vi "interfaz-grafica - Control Mouse.vi"() -> ()   [LabVIEW 2024]
uses:
  TG JD - running/TG Juan Diego/Documentos de Labview/160620 Optotune Lens Driver 4 Labview package/Hello Optotune Lens (30.06.2015)/Calibration.ctl
  <vilib>/vision/Avi.llb/IMAQ AVI2 Refnum.ctl
  <vilib>/Instr/_visa.llb/VISA Configure Serial Port (Instr).vi
  <vilib>/Utility/file.llb/Write Delimited Spreadsheet (string).vi
  <vilib>/Utility/file.llb/Read Delimited Spreadsheet (string).vi
  <vilib>/Utility/inputDevices.llb/mouseAcquire.vi
  <vilib>/Utility/inputDevices.llb/closeMouse.vi
  <vilib>/vision/NI_Vision_Development_Module.lvlib
panel:
  out "Path Pot Inicial IZQUIERDA":path
  out "Path Pot Inicial DERECHA":path
  out "PI_I":dbl(slide) scale=-3.0..3.0
  out "PI_D":dbl(slide) scale=-3.0..3.0
  in  "stop 7":bool
  in  "CONTROL":bool
  out "axis info":T1
  in  "stop 6":bool
  out "Vertical":i32
  out "Dioptrias Finales":dbl
  out "AVI Refnum":T2
  in  "stop 5":bool
  out "Boolean":bool
  out "Usuario 3":string(combo)
  out "Usuario 2":string(combo)
  out "USUARIO 2":string caption="USUARIO"
  out "Path Video":path
  out "Path Potencia Optica D":path
  out "Path Potencia Optica I":path
  in  "stop":bool
  out "Array 2":dbl[](array[numeric])
  out "Array":dbl[](array[numeric])
  out "Path DATOS":path
  in  "stop 2":bool
  out "Path":path=path "C:/Users/willi/GITHUB/TG/OBJ 2 - RECOLECCION DE DATOS/registro-usuarios.csv"
  out "error out":errorcluster
  in  "Tab Control":enum32{"Experimento", "Configuración"}(tab)
  in  "ADQUIRIR":bool
  in  "DETENER":bool
  out "DPT  IZQ":dbl
  out "DPT  DER":dbl
  out "Potencia  Ojo Derecho":dbl[](graph)
  out "ROI (Ojo)":T3(plugin-control)
  out "Path ADQUISICION":path
  in  "Potencia inicial lente derecho":dbl(slide) scale=-3.0..3.0
  in  "Potencia inicial lente izquierdo":dbl(slide) scale=-3.0..3.0
  out "Full Image":T3(plugin-control)
  in  "VISA resource name 3":refnum<visa-resource-name>
  in  "Tab Control 2":T4(tab)
  in  "Usuario":string(combo)
  in  "registrarButtom":bool
  in  "Cluster":T5 {"Fecha de nacimiento" format="%<%x>T"}
  out "Nuevo Usuario":i32
  out "USUARIO":string
  in  "VISA resource name 4":refnum<visa-resource-name>
  out "error out 4":errorcluster
  out "error out 3":errorcluster
  in  "stop 4":bool
  in  "error in (no error) 3":errorcluster
  in  "error in (no error) 4":errorcluster
  in  "stop 3":bool
  out "VISA resource name out 2":string
  out "Command to Port":string
  out "Data":string
  out "OK":bool
  out "Calibration 2":T6 {"Max Current A" format="%#_g mA"; "Max Current B" format="%#_g mA"; "UCL A" format="%#_g mA"; "LCL A" format="%#_g mA"; "UCL B" format="%#_g mA"; "LCL B" format="%#_g mA"}
  out "VISA resource name out":string
  out "ID":u16
  in  "Calibration":T6={"Max Current A"=293.0, "Max Current B"=293.0, "UCL A"=300.0, "UCL B"=300.0, "LCL A"=0.0, "LCL B"=0.0} {"Max Current A" format="%#_g mA"; "Max Current B" format="%#_g mA"; "UCL A" format="%#_g mA"; "LCL A" format="%#_g mA"; "UCL B" format="%#_g mA"; "LCL B" format="%#_g mA"}
  # "Seleccione la Region de Interes (ROI. el ojo)"
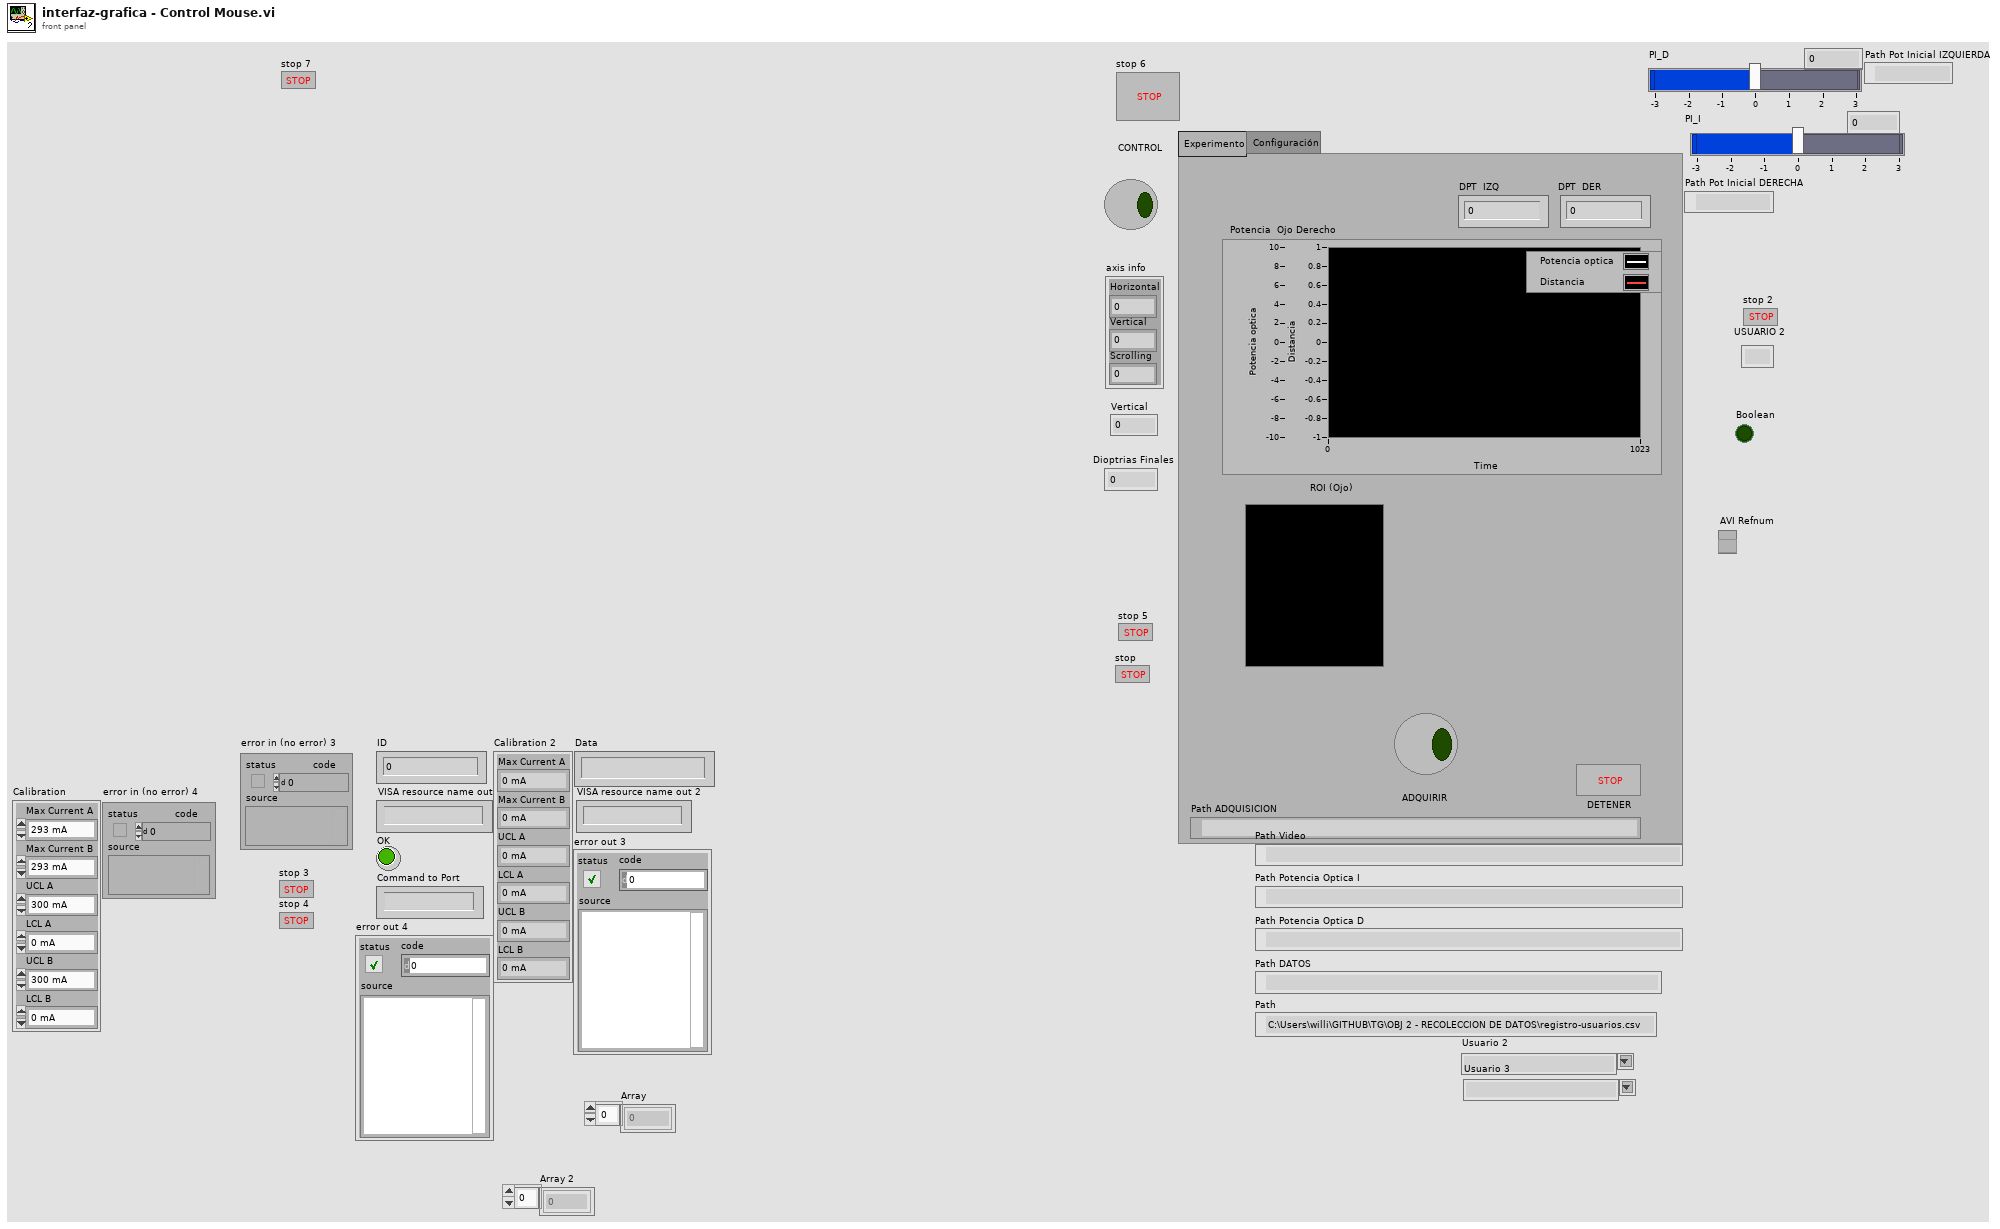
[diagram p1: front panel]
types:
  T1 = cluster{"Horizontal":i32, "Vertical":i32, "Scrolling":i32}
  T2 = typedef "IMAQ AVI2 Refnum.ctl" = refnum<k20>
  T3 = typedef "IMAQ Image.ctl" = refnum<image>
  T4 = enum32{"Seleccionar Usuario", "Registrar Nuevo Usuario"}
  T5 = cluster{"Fecha de nacimiento":timestamp, "Genero":enum16{"Mujer", "Hombre"}, "Error Refractivo":enum16{"No sabe", "Miopia", "Hipermetropia", "No tiene"}}
  T6 = typedef "Calibration.ctl" = cluster{"Max Current A":dbl, "Max Current B":dbl, "UCL A":dbl, "UCL B":dbl, "LCL A":dbl, "LCL B":dbl}
  T7 = typedef "Image Type" = u32
  T8 = cluster{"Global Rectangle":i32[], "Contours":cluster{"Contour Type":u32, "ROI Type":u32, "Points":i32[]}[]}
  T9 = cluster{"Numero \nUsuario":i32, "Fecha de nacimiento":timestamp, "Genero":enum16{"Mujer", "Hombre"}, "Error Refractivo":enum16{"No sabe", "Miopia", "Hipermetropia", "No tiene"}}
  T10 = enum16{"No sabe", "Miopia", "Hipermetropia", "No tiene"}
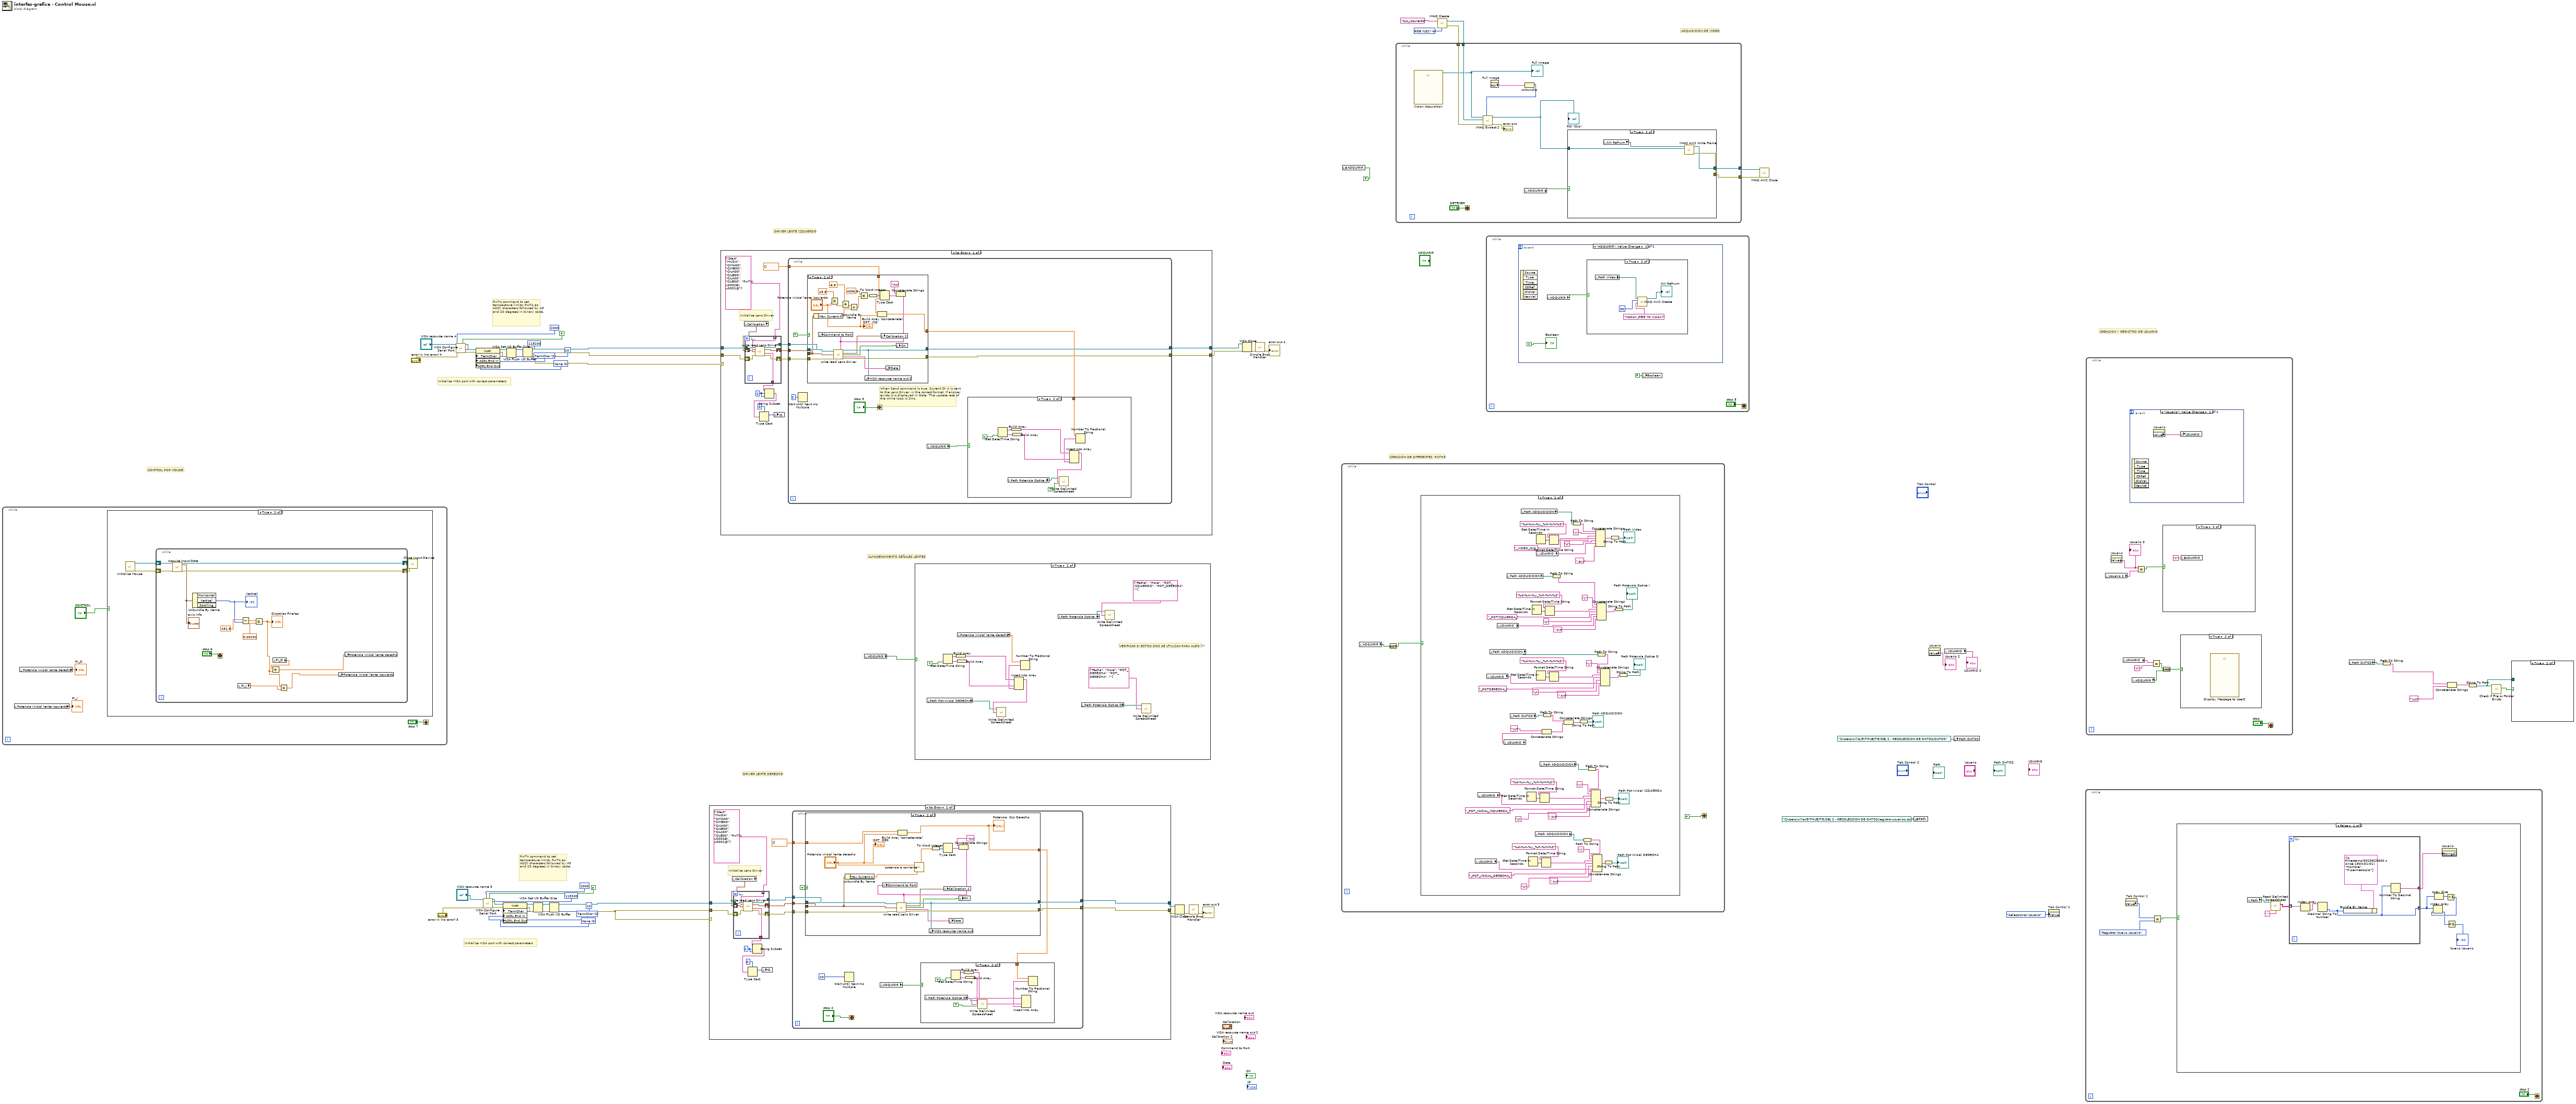
[diagram p0: block diagram]
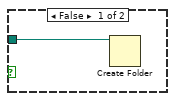
[diagram p4: hidden frame]
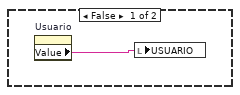
[diagram p6: hidden frame]
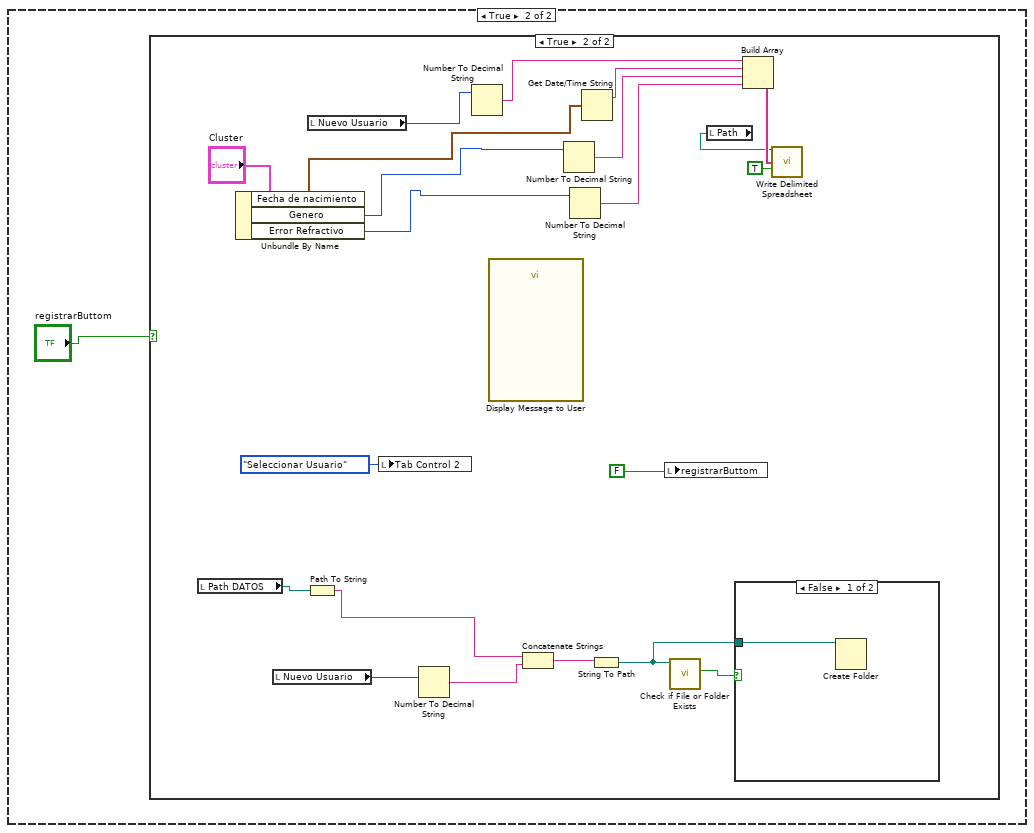
[diagram p9: hidden frame]
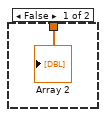
[diagram p13: hidden frame]
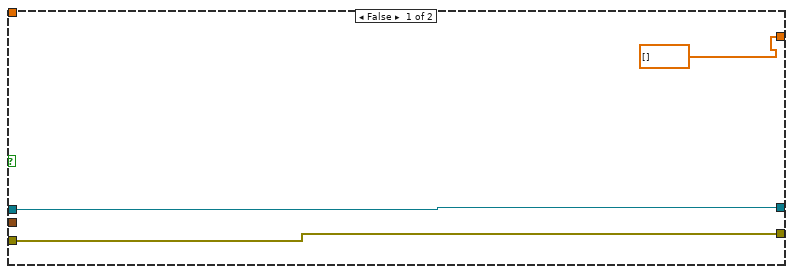
[diagram p14: hidden frame]
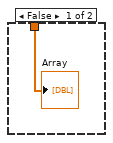
[diagram p16: hidden frame]
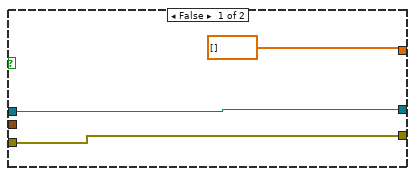
[diagram p17: hidden frame]
diagram:
  w20 = T7 4 items=["Grayscale (U8)", "Grayscale (I16)", "Grayscale (SGL)", "Complex (CSG)", "RGB (U32)", "HSL (U32)", "RGB (U64)", "Grayscale (U16)"] ("Image Type")
  w41 = u16 0 items=["None", "Last Bit", "TermChar", "Break"] ("Serial Settings:End Mode for Writes")
  w40 = u16 2 items=["None", "Last Bit", "TermChar"] ("Serial Settings:End Mode for Reads")
  w53 = u16 0 items=["None", "Last Bit", "TermChar", "Break"] ("Serial Settings:End Mode for Writes")
  w52 = u16 2 items=["None", "Last Bit", "TermChar"] ("Serial Settings:End Mode for Reads")
  # "ADQUISICIÓN DE VIDEO"
  # "CREACION Y REGISTRO DE USUARIO"
  # "CREACIÓN DE DIFERENTES 'PATHS'"
  # "ALMACENAMIENTO SEÑALES LENTES"
  # "DRIVER LENTE DERECHO"
  # "DRIVER LENTE IZQUIERDO"
  # "CONTROL POR MOUSE"
  # "PwTA command to set temperature limits: PwTA as ASCII characters followed by 45 and 20 degrees in binary code."
  # "Initialize VISA port with correct parameters"
  # "PwTA command to set temperature limits: PwTA as ASCII characters followed by 45 and 20 degrees in binary code."
  # "Initialize VISA port with correct parameters"
  n1 = while {
    stop <- "stop 7" stop-if-true
    n2 = local read "Potencia inicial lente izquierdo"() -> (→"PI_I":dbl)
    n3 = local read "Potencia inicial lente derecho"() -> (→"PI_D":dbl)
    n4 = case shown="True" "CONTROL" {
      frame False {
      }
      frame True {
        n5 = call <vilib>:"Initialize Mouse.vi"() -> ("error out"=w65:errorcluster, "device ID"=w67:refnum<k1>)  [unwired: 10 in]
        n6 = while {
          shift-right: [w81] -> w66
          shift-left: w67 -> [w82]
          shift-right: [w79] -> w64
          shift-left: w65 -> [w80]
          stop <- "stop 6" stop-if-true
          n7 = call-poly <vilib>:"Acquire Input Data.vi"("device ID"=w82, "error in (no error)"=w80) -> ("device ID"=w81:refnum<k1>, "axis info"=w77:T1, "error out"=w79:errorcluster)  [unwired: 14 in, 1 out]
          "axis info" <- w77
          n8 = Unbundle By Name(w77) -> ("Vertical"=w76:i32)  [unwired: 2 out]
          "Vertical" <- w76
          n9 = local read "PI_I"() -> (w72:dbl)
          n10 = Subtract(x=431.5, y=w76) -> (x-y=w74:dbl)
          n11 = Multiply(x=w74, y=0.00232) -> (x*y=w70:dbl)
          "Dioptrias Finales" <- w70
          n12 = local read "PI_D"() -> (w71:dbl)
          n13 = Add(x=w71, y=w70) -> (x+y=w69:dbl)
          n14 = Add(x=w70, y=w72) -> (x+y=w68:dbl)
          n15 = local write "Potencia inicial lente izquierdo"(w68) -> ()
          n16 = local write "Potencia inicial lente derecho"(w69) -> ()
        }
        n17 = call-poly <vilib>:"Close Input Device.vi"("error in (no error)"=w64, "device ID"=w66) -> ()  [unwired: 8 in, 1 out]
      }
    }
  }
  n18 = call-poly "VISA Configure Serial Port"("VISA resource name"="VISA resource name 4", "timeout (10sec)"=u32 2000, "Enable Termination\nChar (T)"=FALSE ("Enable Termination\nChar (T)"), "baud rate (9600)"=u32 115200, "error in (no error)"="error in (no error) 4") -> ("VISA resource name out"=w48:refnum<visa-resource-name>, "error out"=w50:errorcluster)  [unwired: 9 in]
  n19 = property class="Instr"(reference=w48, error in=w50, "TermChar"=u8 10 ("Message Based Settings:Termination Character"), "ASRL End In"=w52, "ASRL End Out"=w53) -> (reference out=w49:refnum<visa-resource-name>, error out=w51:errorcluster)
  n20 = call-poly "VISA Configure Serial Port"("VISA resource name"="VISA resource name 3", "timeout (10sec)"=u32 2000, "Enable Termination\nChar (T)"=FALSE ("Enable Termination\nChar (T)"), "baud rate (9600)"=u32 115200, "error in (no error)"="error in (no error) 3") -> ("VISA resource name out"=w36:refnum<visa-resource-name>, "error out"=w38:errorcluster)  [unwired: 9 in]
  n21 = property class="Instr"(reference=w36, error in=w38, "TermChar"=u8 10 ("Message Based Settings:Termination Character"), "ASRL End In"=w40, "ASRL End Out"=w41) -> (reference out=w37:refnum<visa-resource-name>, error out=w39:errorcluster)
  n22 = VISA Set I/O Buffer Size(VISA resource name=w49, error in (no error)=w51) -> (VISA resource name out=w55:refnum<visa-resource-name>, error out=w56:errorcluster)  [unwired: 2 in]
  n23 = VISA Flush I/O Buffer(VISA resource name=w55, error in (no error)=w56) -> (VISA resource name out=w58:refnum<visa-resource-name>, error out=w57:errorcluster)  [unwired: 1 in]
  n24 = VISA Set I/O Buffer Size(VISA resource name=w37, error in (no error)=w39) -> (VISA resource name out=w43:refnum<visa-resource-name>, error out=w44:errorcluster)  [unwired: 2 in]
  n25 = VISA Flush I/O Buffer(VISA resource name=w43, error in (no error)=w44) -> (VISA resource name out=w31:refnum<visa-resource-name>, error out=w30:errorcluster)  [unwired: 1 in]
  n26 = case shown="No Error" w30 {
    tunnel: w30 -> [w97 w148]
    tunnel: w31 -> [w96 w149]
    tunnel: [w95 w148] -> w26
    tunnel: [w94 w149] -> w27
    frame No Error {
      w93 = 2 ("length (rest)")
      # "Initialize Lens Driver"
      n27 = local read "Calibration"() -> (w85:T6)
      n28 = for {
        tunnel: w96 -> [w146]
        tunnel: [w143] -> w88
        tunnel: string[] ["Start", "MwDA", "CrMA00", "CrMB00", "CrUA00", "CrUB00", "CrLA00", "CrLB00", "PwTA\u0002Ð\u0001@"] -> [w141] mode=indexing
        tunnel: [w140] -> w87
        shift-right: [w144] -> w89
        shift-left: w85 -> [w145]
        shift-right: [w142] -> w90
        shift-left: w97 -> [w147]
        n29 = call "write read Lens Driver.vi"("VISA resource name"=w146, "command"=w141, "Calibration"=w145, "error in (no error)"=w147) -> ("VISA resource name out"=w143:refnum<visa-resource-name>, "Calibration 2"=w144:T6, "Data"=w140:string, "error out"=w142:errorcluster)  [unwired: 4 in, 4 out]
      }
      n30 = String Subset(string=w87, offset (0)=w93, length (rest)=w93) -> (substring=w91:string)
      n31 = Type Cast(type=u16 0 ("length (rest)"), x=w91) -> (*(type *) &x=w86:u16)
      n32 = local write "ID"(w86) -> ()
      n33 = while {
        tunnel: [w102] -> w95
        tunnel: [w103] -> w94
        tunnel: w90 -> [w108]
        tunnel: w89 -> [w107]
        tunnel: w88 -> [w106]
        tunnel: dbl[] [] -> [w100]
        stop <- "stop 4" stop-if-true
        n34 = case shown="True" TRUE ("Send command") {
          tunnel: [w122 w139] -> w102
          tunnel: w108 -> [w122 w138]
          tunnel: w107 -> [_ w129]
          tunnel: w106 -> [w121 w137]
          tunnel: [w121 w130] -> w103
          tunnel: w100 -> [_ w124]
          tunnel: [dbl[] [] w123] -> w99
          frame False {
          }
          frame True {
            n35 = Unbundle By Name(w129) -> ("Max Current A"=w128:dbl)
            n36 = Build Array (concatenate)(w124, "Potencia inicial lente derecho") -> (w123:dbl[])
            "Potencia  Ojo Derecho" <- w123
            n37 = call "potencia a corriente.vi"("Max current A"=w128, "Potencia"="Potencia inicial lente derecho") -> ("Corriente"=w127:dbl)
            n38 = To Word Integer(number=w127) -> (16bit integer=w136:i16)
            n39 = Type Cast(x=w136) -> (*(type *) &x=w135:string)  [unwired: 1 in]
            n40 = Concatenate Strings("Aw", w135) -> (w132:string)
            n41 = local write "Command to Port"(w132) -> ()
            n42 = call "write read Lens Driver.vi"("VISA resource name"=w137, "command"=w132, "Calibration"=w129, "error in (no error)"=w138) -> ("VISA resource name out"=w130:refnum<visa-resource-name>, "Calibration 2"=w134:T6, "OK"=w133:bool, "Data"=w131:string, "error out"=w139:errorcluster)  [unwired: 4 in, 3 out]
            n43 = local write "VISA resource name out"(w130) -> ()
            n44 = local write "Calibration 2"(w134) -> ()
            n45 = local write "Data"(w131) -> ()
            n46 = local write "OK"(w133) -> ()
            "DPT  DER" <- "Potencia inicial lente derecho"
          }
        }
        n47 = Wait Until Next ms Multiple(millisecond multiple=u32 20) -> ()  [unwired: 1 out]
        n48 = local read "ADQUIRIR"() -> (w98:bool)
        n49 = case shown="True" w98 {
          tunnel: w99 -> [w109 w111]
          frame False {
            "Array 2" <- w109
          }
          frame True {
            n50 = local read "Path Potencia Optica D"() -> (w110:path)
            n51 = Get Date/Time String(want seconds? (F)=TRUE) -> (date string=w119:string, time string=w118:string)  [unwired: 2 in]
            n52 = Build Array(w119) -> (w117:string[])
            n53 = Build Array(w118) -> (w116:string[])
            n54 = Number To Fractional String(number=w111) -> (F-format string=w112:string[])  [unwired: 3 in]
            n55 = Insert Into Array(array=w117, new element #1=w116, new element #2=w112) -> (w115:string[])  [unwired: 1 in]
            n56 = call-poly <vilib>:"Write Delimited Spreadsheet.vi"("file path (dialog if empty)"=w110, "1D data"=w115, "append to file? (new file:F)"=TRUE) -> ()  [unwired: 11 in, 2 out]
          }
        }
      }
    }
    frame Error {
    }
  }
  n57 = case shown="No Error" w57 {
    tunnel: w57 -> [w164 w221]
    tunnel: w58 -> [w163 w222]
    tunnel: [w162 w221] -> w23
    tunnel: [w161 w222] -> w22
    frame No Error {
      w160 = 2 ("length (rest)")
      # "Initialize Lens Driver"
      n58 = local read "Calibration"() -> (w152:T6)
      n59 = for {
        tunnel: w163 -> [w219]
        tunnel: [w216] -> w155
        tunnel: string[] ["Start", "MwDA", "CrMA00", "CrMB00", "CrUA00", "CrUB00", "CrLA00", "CrLB00", "PwTA\u0002Ð\u0001@"] -> [w214] mode=indexing
        tunnel: [w213] -> w154
        shift-right: [w217] -> w156
        shift-left: w152 -> [w218]
        shift-right: [w215] -> w157
        shift-left: w164 -> [w220]
        n60 = call "write read Lens Driver.vi"("VISA resource name"=w219, "command"=w214, "Calibration"=w218, "error in (no error)"=w220) -> ("VISA resource name out"=w216:refnum<visa-resource-name>, "Calibration 2"=w217:T6, "Data"=w213:string, "error out"=w215:errorcluster)  [unwired: 4 in, 4 out]
      }
      n61 = String Subset(string=w154, offset (0)=w160, length (rest)=w160) -> (substring=w158:string)
      n62 = Type Cast(type=u16 0 ("length (rest)"), x=w158) -> (*(type *) &x=w153:u16)
      n63 = local write "ID"(w153) -> ()
      n64 = while {
        tunnel: [w169] -> w162
        tunnel: [w170] -> w161
        tunnel: w157 -> [w175]
        tunnel: w156 -> [w174]
        tunnel: w155 -> [w173]
        tunnel: dbl[] [] -> [w166]
        stop <- "stop 3" stop-if-true
        # "When Send command is true, Current Ch A is sent to the Lens Driver, in the correct format. If answer exists it is displayed in Data. The update rate of the while loop is 2ms."
        n65 = Wait Until Next ms Multiple(millisecond multiple=u32 2) -> ()  [unwired: 1 out]
        n66 = case shown="True" TRUE ("Send command") {
          tunnel: [w189 w212] -> w169
          tunnel: w175 -> [w189 w211]
          tunnel: w174 -> [_ w199]
          tunnel: w173 -> [w188 w210]
          tunnel: [w188 w200] -> w170
          tunnel: [dbl[] [] w190] -> w167
          tunnel: w166 -> [_ w192]
          frame False {
          }
          frame True {
            n67 = Unbundle By Name(w199) -> ("Max Current A"=w198:dbl)
            n68 = Multiply(x=15.8, y="Potencia inicial lente izquierdo") -> (x*y=w196:dbl)
            n69 = Add(x=-6.8, y=w196) -> (x+y=w194:dbl)
            n70 = Divide(x=w194, y=w198) -> (x/y=w197:dbl)
            n71 = Multiply(x=4096.0, y=w197) -> (x*y=w208:dbl)
            n72 = To Word Integer(number=w208) -> (16bit integer=w207:i16)
            n73 = Build Array (concatenate)(w192, "Potencia inicial lente izquierdo") -> (w190:dbl[])
            n74 = Type Cast(x=w207) -> (*(type *) &x=w206:string)  [unwired: 1 in]
            n75 = Concatenate Strings("Aw", w206) -> (w202:string)
            n76 = local write "Command to Port"(w202) -> ()
            n77 = call "write read Lens Driver.vi"("VISA resource name"=w210, "command"=w202, "Calibration"=w199, "error in (no error)"=w211) -> ("VISA resource name out"=w200:refnum<visa-resource-name>, "Calibration 2"=w204:T6, "OK"=w203:bool, "Data"=w201:string, "error out"=w212:errorcluster)  [unwired: 4 in, 3 out]
            n78 = local write "VISA resource name out 2"(w200) -> ()
            n79 = local write "Calibration 2"(w204) -> ()
            n80 = local write "Data"(w201) -> ()
            n81 = local write "OK"(w203) -> ()
            "DPT  IZQ" <- "Potencia inicial lente izquierdo"
          }
        }
        n82 = local read "ADQUIRIR"() -> (w165:bool)
        n83 = case shown="True" w165 {
          tunnel: w167 -> [w176 w178]
          frame False {
            "Array" <- w176
          }
          frame True {
            n84 = Get Date/Time String(want seconds? (F)=TRUE) -> (date string=w186:string, time string=w185:string)  [unwired: 2 in]
            n85 = local read "Path Potencia Optica I"() -> (w177:path)
            n86 = Build Array(w186) -> (w184:string[])
            n87 = Build Array(w185) -> (w183:string[])
            n88 = Number To Fractional String(number=w178) -> (F-format string=w179:string[])  [unwired: 3 in]
            n89 = Insert Into Array(array=w184, new element #1=w183, new element #2=w179) -> (w182:string[])  [unwired: 1 in]
            n90 = call-poly <vilib>:"Write Delimited Spreadsheet.vi"("file path (dialog if empty)"=w177, "1D data"=w182, "append to file? (new file:F)"=TRUE) -> ()  [unwired: 11 in, 2 out]
          }
        }
      }
    }
    frame Error {
    }
  }
  n91 = local read "ADQUIRIR"() -> (w12:bool)
  n92 = case shown="True" w12 {
    frame False {
    }
    frame True {
      # "VERIFICAR SI ESTOS DOS SE UTILIZAN PARA ALGO (?)"
      n93 = local read "Path Pot Inicial DERECHA"() -> (w223:path)
      n94 = Get Date/Time String(want seconds? (F)=TRUE) -> (date string=w231:string, time string=w230:string)  [unwired: 2 in]
      n95 = Build Array(w231) -> (w229:string[])
      n96 = local read "Potencia inicial lente derecho"() -> (w225:dbl)
      n97 = Build Array(w230) -> (w228:string[])
      n98 = Number To Fractional String(number=w225) -> (F-format string=w226:string)  [unwired: 3 in]
      n99 = Insert Into Array(array=w229, new element #1=w228, new element #2=w226) -> (w224:string[])  [unwired: 1 in]
      n100 = call-poly <vilib>:"Write Delimited Spreadsheet.vi"("file path (dialog if empty)"=w223, "1D data"=w224) -> ()  [unwired: 12 in, 2 out]
      n101 = local read "Path Potencia Optica I"() -> (w233:path)
      n102 = local read "Path Potencia Optica D"() -> (w232:path)
      n103 = call-poly <vilib>:"Write Delimited Spreadsheet.vi"("file path (dialog if empty)"=w233, "1D data"=string[] ["Fecha", "Hora", "POT_IZQUIERDO", "POT_DERECHA", ""]) -> ()  [unwired: 12 in, 2 out]
      n104 = call-poly <vilib>:"Write Delimited Spreadsheet.vi"("file path (dialog if empty)"=w232, "1D data"=string[] ["Fecha", "Hora", "POT_DERECHA", "POT_DERECHA", ""]) -> ()  [unwired: 12 in, 2 out]
    }
  }
  n105 = VISA Close(VISA resource name=w27, error in (no error)=w26) -> (error out=w29:errorcluster)
  n106 = call <vilib>:"Simple Error Handler.vi"("error in (no error)"=w29) -> ("error out"=→"error out 3":errorcluster)  [unwired: 4 in, 4 out]
  n107 = VISA Close(VISA resource name=w22, error in (no error)=w23) -> (error out=w25:errorcluster)
  n108 = call <vilib>:"Simple Error Handler.vi"("error in (no error)"=w25) -> ("error out"=→"error out 4":errorcluster)  [unwired: 4 in, 4 out]
  n109 = while {
    stop <- FALSE ("stop 5") stop-if-true
    n110 = local read "ADQUIRIR"() -> (w237:bool)
    n111 = Not(x=w237) -> (.not. x?=w236:bool)
    n112 = case shown="True" w236 {
      frame False {
      }
      frame True {
        n113 = local read "USUARIO"() -> (w245:string)
        n114 = local read "USUARIO"() -> (w246:string)
        n115 = local read "USUARIO"() -> (w298:string)
        n116 = local read "Path ADQUISICION"() -> (w295:path)
        n117 = local read "USUARIO"() -> (w297:string)
        n118 = local read "USUARIO"() -> (w279:string)
        n119 = local read "Path ADQUISICION"() -> (w296:path)
        n120 = local read "Path DATOS"() -> (w280:path)
        n121 = local read "Path ADQUISICION"() -> (w305:path)
        n122 = Get Date/Time In Seconds() -> (seconds since 1Jan1904=w261:timestamp)
        n123 = Get Date/Time In Seconds() -> (seconds since 1Jan1904=w254:timestamp)
        n124 = Get Date/Time In Seconds() -> (seconds since 1Jan1904=w285:timestamp)
        n125 = local read "Path ADQUISICION"() -> (w243:path)
        n126 = Get Date/Time In Seconds() -> (seconds since 1Jan1904=w300:timestamp)
        n127 = Get Date/Time In Seconds() -> (seconds since 1Jan1904=w288:timestamp)
        n128 = local read "USUARIO"() -> (w302:string)
        n129 = Format Date/Time String(time format string (%c)="%d-%m-%y_%H-%M-%S", seconds (now)=w261) -> (date/time string=w262:string)  [unwired: 1 in]
        n130 = local read "Path ADQUISICION"() -> (w256:path)
        n131 = Format Date/Time String(time format string (%c)="%d-%m-%y_%H-%M-%S", seconds (now)=w254) -> (date/time string=w255:string)  [unwired: 1 in]
        n132 = Path To String(path=w280) -> (string=w281:string)
        n133 = Concatenate Strings("\\U" ("string"), w279) -> (w282:string)
        n134 = Format Date/Time String(time format string (%c)="%d-%m-%y_%H-%M-%S", seconds (now)=w285) -> (date/time string=w287:string)  [unwired: 1 in]
        n135 = Format Date/Time String(time format string (%c)="%d-%m-%y_%H-%M-%S", seconds (now)=w300) -> (date/time string=w301:string)  [unwired: 1 in]
        n136 = Format Date/Time String(time format string (%c)="%d-%m-%y_%H-%M-%S", seconds (now)=w288) -> (date/time string=w290:string)  [unwired: 1 in]
        n137 = Path To String(path=w296) -> (string=w291:string)
        n138 = Concatenate Strings(w281, w282) -> (w283:string)
        n139 = Path To String(path=w305) -> (string=w299:string)
        n140 = String To Path(string=w283) -> (path=→"Path ADQUISICION":path)
        n141 = Path To String(path=w243) -> (string=w244:string)
        n142 = Path To String(path=w256) -> (string=w257:string)
        n143 = Concatenate Strings(w257, "\\" ("string"), w262, "_POT_INICIAL_IZQUIERDA_" ("string"), "U" ("string"), w246, ".txt" ("string")) -> (w242:string)
        n144 = Concatenate Strings(w244, "\\" ("string"), w255, "_POT_INICIAL_DERECHA_" ("string"), "U" ("string"), w245, ".txt" ("string")) -> (w241:string)
        n145 = Concatenate Strings(w299, "\\" ("string"), w301, "_VIDEO_OJO_" ("string"), "U" ("string"), w302, ".avi" ("string")) -> (w303:string)
        n146 = Concatenate Strings(w291, "\\" ("string"), w287, "_POTIZQUIERDA_" ("string"), "U" ("string"), w297, ".txt" ("string")) -> (w286:string)
        n147 = Path To String(path=w295) -> (string=w292:string)
        n148 = Concatenate Strings(w292, "\\" ("string"), w290, "_POTDERECHA_" ("string"), "U" ("string"), w298, ".txt" ("string")) -> (w289:string)
        n149 = String To Path(string=w241) -> (path=→"Path Pot Inicial DERECHA":path)
        n150 = String To Path(string=w242) -> (path=→"Path Pot Inicial IZQUIERDA":path)
        n151 = String To Path(string=w303) -> (path=→"Path Video":path)
        n152 = String To Path(string=w286) -> (path=→"Path Potencia Optica I":path)
        n153 = String To Path(string=w289) -> (path=→"Path Potencia Optica D":path)
      }
    }
  }
  n154 = local write "ADQUIRIR"(FALSE ("ADQUIRIR")) -> ()
  n155 = call "IMAQ Create"("Image Name"="ojo_izquierdo", "Image Type"=w20) -> ("New Image"=w18:T3, "error out"=w19:errorcluster)  [unwired: 3 in]
  n156 = while {
    tunnel: w19 -> [w315]
    tunnel: w18 -> [w314]
    tunnel: [w308] -> w17
    tunnel: [w307] -> w16
    stop <- "DETENER" stop-if-true
    n157 = call "Vision Acquisition"() -> ("Image Out"=w310:T3)  [unwired: 25 in, 2 out]
    "Full Image" <- w310
    n158 = property on="Full Image" class="ImageControl"() -> ("ROI"=w313:T8)  [unwired: 2 in, 2 out]
    n159 = local read "ADQUIRIR"() -> (w306:bool)
    n160 = Unbundle "Unbundle"(w313) -> ("Global Rectangle"=w312:i32[])  [unwired: 1 out]
    n161 = call "IMAQ Extract 2"("Optional Rectangle"=w312, "error in (no error)"=w315, "Image Dst"=w314, "Image Src"=w310) -> ("error out"=→"error out":errorcluster, "Image Dst Out"=w309:T3)  [unwired: 6 in]
    "ROI (Ojo)" <- w309
    n162 = case shown="True" w306 {
      tunnel: [_ w320] -> w308
      tunnel: [_ w319] -> w307
      tunnel: w309 -> [_ w318]
      frame False {
      }
      frame True {
        n163 = local read "AVI Refnum"() -> (w317:T2)
        n164 = call "IMAQ AVI2 Write Frame"("Image"=w318, "AVI Refnum"=w317) -> ("error out"=w320:errorcluster, "AVI Refnum (duplicate)"=w319:T2)  [unwired: 7 in, 1 out]
      }
    }
  }
  n165 = while {
    stop <- "stop 5" stop-if-true
    n166 = event shown="[0] \"ADQUIRIR\": Value Change" {
      selector: _ -> [_]
      dyn-events: _ -> [_]
      timeout: _ -> [_]
      event "ADQUIRIR": Value Change {
        n167 = event-data() -> ()  [unwired: 1 in, 6 out]
        n168 = local read "ADQUIRIR"() -> (w323:bool)
        n169 = case shown="True" w323 {
          frame False {
          }
          frame True {
            n170 = local read "Path Video"() -> (w327:path)
            n171 = call "IMAQ AVI2 Create"("Codec"="Motion JPEG (NI Vision)", "Frames Per Second"=u32 30, "AVI Path"=w327) -> ("AVI Refnum"=→"AVI Refnum":T2)  [unwired: 7 in, 1 out]
          }
        }
        "Boolean" <- TRUE
      }
    }
    n172 = local write "Boolean"(FALSE ("Boolean")) -> ()
  }
  n173 = call "IMAQ AVI2 Close"("error in (no error)"=w17, "AVI Refnum"=w16) -> ()  [unwired: 9 in, 1 out]
  n174 = local write "Path"(path "C:/Users/willa/GITHUB/TG/OBJ 2 - RECOLECCION DE DATOS/registro-usuarios.csv" ("Path")) -> ()
  n175 = property on="Usuario" class="CmbBox"() -> ("Value"=→"Usuario 2":string)  [unwired: 2 in, 2 out]
  n176 = local read "USUARIO"() -> (→"USUARIO 2":string)
  n177 = local write "Path DATOS"(path "C:/Users/willa/GITHUB/TG/OBJ 2 - RECOLECCION DE DATOS/DATOS" ("Path DATOS")) -> ()
  n178 = property on="Tab Control 2" class="TabCtl (strict)"("Value"=T4."Seleccionar Usuario" ("Tab Control 2")) -> ()  [unwired: 2 in, 2 out]
  n179 = while {
    stop <- "stop 2" stop-if-true
    n180 = property on="Tab Control 2" class="TabCtl (strict)"() -> ("Value"=w331:T4)  [unwired: 2 in, 2 out]
    n181 = Equal?(x=w331, y=T4."Registrar Nuevo Usuario") -> (x = y?=w332:bool)
    n182 = case shown="False" w332 {
      frame False {
        n183 = local read "Path"() -> (w340:path)
        n184 = call-poly <vilib>:"Read Delimited Spreadsheet.vi"("file path (dialog if empty)"=w340, "delimiter (\\t)"="," ("delimiter (\\t)")) -> ("all rows"=w339:string[][])  [unwired: 8 in, 5 out]
        n185 = for {
          tunnel: w339 -> [w346] mode=indexing
          tunnel: [w343] -> w338 mode=indexing
          tunnel: [w342] -> w333 mode=indexing
          n186 = Index Array(array=w346) -> (element=w344:string)  [unwired: 1 in]
          n187 = Decimal String To Number(string=w344) -> (number=w343:i32)  [unwired: 2 in, 1 out]
          n188 = Bundle By Name(cluster=T9 {"Numero \nUsuario"=0, "Fecha de nacimiento"=timestamp(3029529600 s since 1904-01-01), "Genero"=enum."Hombre", "Error Refractivo"=enum."Hipermetropia"} ("Cluster"), "Numero \nUsuario"=w343) -> ()  [unwired: 1 out]
          n189 = Number To Decimal String(number=w343) -> (decimal integer string=w342:string)  [unwired: 1 in]
        }
        n190 = Array Size(array=w338) -> (size(s)=w337:i32)
        n191 = property on="Usuario" class="CmbBox"("Strings[]"=w333) -> ()  [unwired: 2 in, 2 out]
        n192 = Decrement(x=w337) -> (x-1=w336:i32)
        n193 = Index Array(array=w338, index=w336) -> (element=w335:i32)
        n194 = Increment(x=w335) -> (x+1=→"Nuevo Usuario":i32)
      }
      frame True {
        n195 = case shown="True" "registrarButtom" {
          frame False {
          }
          frame True {
            n196 = local read "Path DATOS"() -> (w349:path)
            n197 = Unbundle By Name("Cluster") -> ("Fecha de nacimiento"=w358:timestamp, "Genero"=w357:enum16{"Mujer", "Hombre"}, "Error Refractivo"=w356:T10)
            n198 = local read "Nuevo Usuario"() -> (w354:i32)
            n199 = Path To String(path=w349) -> (string=w348:string)
            n200 = local read "Nuevo Usuario"() -> (w355:i32)
            n201 = local write "Tab Control 2"(T4."Seleccionar Usuario" ("Tab Control 2")) -> ()
            n202 = Number To Decimal String(number=w354) -> (decimal integer string=w353:string)  [unwired: 1 in]
            n203 = Number To Decimal String(number=w355) -> (decimal integer string=w363:string)  [unwired: 1 in]
            n204 = call "Display Message to User"() -> ()  [unwired: 10 in, 2 out]
            n205 = Concatenate Strings(w348, w353) -> (w352:string)
            n206 = Number To Decimal String(number=w357) -> (decimal integer string=w361:string)  [unwired: 1 in]
            n207 = Number To Decimal String(number=w356) -> (decimal integer string=w360:string)  [unwired: 1 in]
            n208 = Get Date/Time String(seconds (now)=w358) -> (date string=w362:string)  [unwired: 2 in, 1 out]
            n209 = String To Path(string=w352) -> (path=w351:path)
            n210 = local write "registrarButtom"(FALSE ("registrarButtom")) -> ()
            n211 = call <vilib>:"Check if File or Folder Exists.vi"("path"=w351) -> ("file or folder exists?"=w350:bool)  [unwired: 8 in, 2 out]
            n212 = local read "Path"() -> (w367:path)
            n213 = case shown="False" w350 {
              tunnel: w351 -> [w369 _]
              frame False {
                n214 = Create Folder(path (use dialog)=w369) -> ()  [unwired: 2 in, 3 out]
              }
              frame True {
              }
            }
            n215 = Build Array(w363, w362, w361, w360) -> (w368:string[])
            n216 = call-poly <vilib>:"Write Delimited Spreadsheet.vi"("file path (dialog if empty)"=w367, "1D data"=w368, "append to file? (new file:F)"=TRUE) -> ()  [unwired: 11 in, 2 out]
          }
        }
      }
    }
  }
  n217 = while {
    stop <- "stop" stop-if-true
    n218 = local read "Usuario 2"() -> (w372:string)
    n219 = property on="Usuario" class="CmbBox"() -> ("Value"=w370:string)  [unwired: 2 in, 2 out]
    "Usuario 3" <- w370
    n220 = local read "USUARIO"() -> (w374:string)
    n221 = event shown="[0] \"Usuario\": Value Change" {
      selector: _ -> [_]
      dyn-events: _ -> [_]
      timeout: _ -> [_]
      event "Usuario": Value Change {
        n222 = event-data() -> ()  [unwired: 1 in, 6 out]
        n223 = property on="Usuario" class="CmbBox"() -> ("Value"=w379:string)  [unwired: 2 in, 2 out]
        n224 = local write "USUARIO"(w379) -> ()
      }
    }
    n225 = local read "ADQUIRIR"() -> (w376:bool)
    n226 = Equal?(x=w370, y=w372) -> (x = y?=w371:bool)
    n227 = Equal?(x=w374, y="X") -> (x = y?=w375:bool)
    n228 = And(x=w375, y=w376) -> (x .and. y?=w377:bool)
    n229 = case shown="True" w371 {
      frame False {
        n230 = property on="Usuario" class="CmbBox"() -> ("Value"=w380:string)  [unwired: 2 in, 2 out]
        n231 = local write "USUARIO"(w380) -> ()
      }
      frame True {
        n232 = local write "USUARIO"("X" ("USUARIO")) -> ()
      }
    }
    n233 = case shown="True" w377 {
      frame False {
      }
      frame True {
        n234 = call "Display Message to User2"() -> ()  [unwired: 10 in, 2 out]
      }
    }
  }
  n235 = local read "Path DATOS"() -> (w4:path)
  n236 = Path To String(path=w4) -> (string=w3:string)
  n237 = Concatenate Strings(w3, "\\UX" ("string")) -> (w7:string)
  n238 = String To Path(string=w7) -> (path=w6:path)
  n239 = call <vilib>:"Check if File or Folder Exists.vi"("path"=w6) -> ("file or folder exists?"=w5:bool)  [unwired: 8 in, 2 out]
  n240 = case shown="True" w5 {
    tunnel: w6 -> [w382 _]
    frame False {
      n241 = Create Folder(path (use dialog)=w382) -> ()  [unwired: 2 in, 3 out]
    }
    frame True {
    }
  }
